vi "csmdoc_export_all_csm_VI_description_doc.vi"(11 "Path":path=path "D:/github/JKI-State-Machine-Plus/.doc/VI Description.md") -> ()   [LabVIEW 2017]
uses:
  Communicable State Machine.lvlib
panel:
  in  "Error in":errorcluster caption="Error in (no error)"
  out "error out":errorcluster
  out "Array":path[](array[path])
  out "concatenated string":string
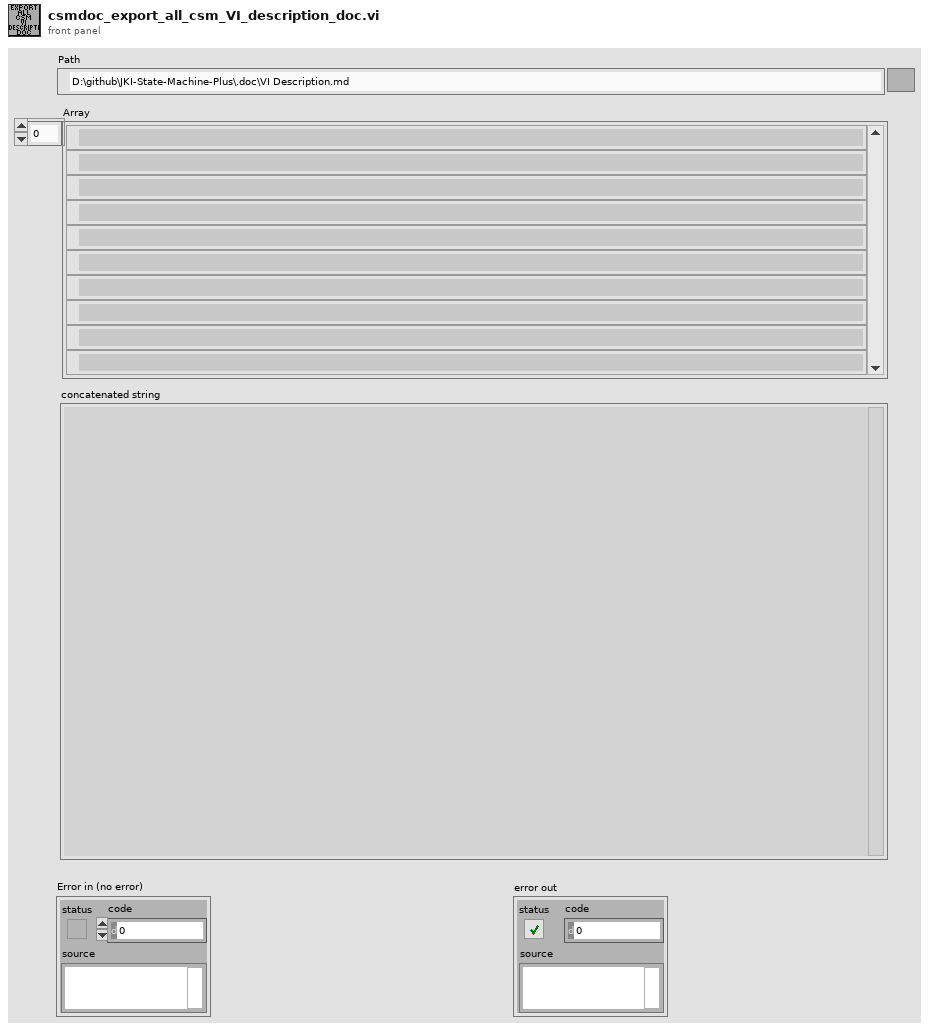
[diagram p1: front panel]
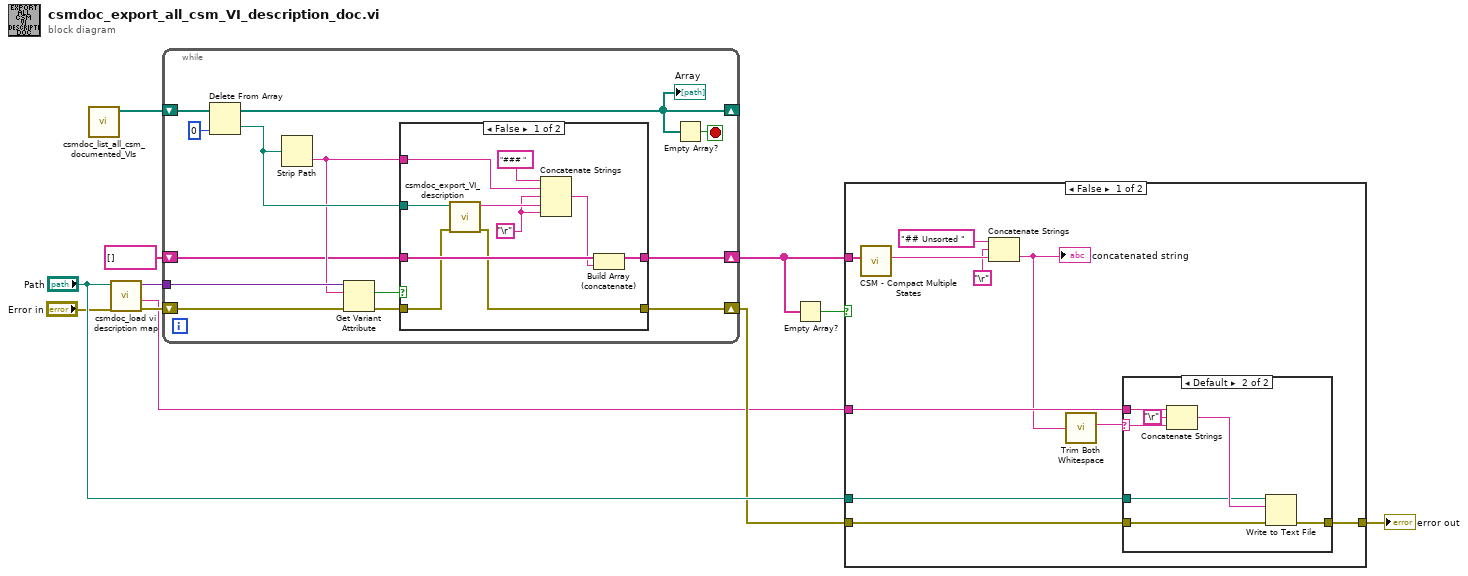
[diagram p0: block diagram]
diagram:
  n1 = call "csmdoc_list_all_csm_documented_VIs.vi"() -> ("Array"=w11:path[])  [unwired: 11 in]
  n2 = call "csmdoc_load vi description map.vi"("Error in"="Error in", "Path"="Path") -> ("Error out"=w7:errorcluster, "text"=w5:string, "variant"=w10:variant)  [unwired: 7 in]
  n3 = while {
    shift-right: [w21] -> _
    shift-left: w11 -> [w23]
    tunnel: w10 -> [w19]
    shift-right: [w16] -> w2
    shift-left: string[] [] -> [w15]
    shift-right: [w12] -> w6
    shift-left: w7 -> [w14]
    stop <- w22 stop-if-true
    n4 = Delete From Array(array=w23, index=0) -> (deleted portion=w24:path, array with subset deleted=w21:path[])  [unwired: 1 in]
    "Array" <- w21
    n5 = Strip Path(path=w24) -> (name=w18:string)  [unwired: 1 out]
    n6 = Get Variant Attribute(Variant=w19, name=w18, error in=w14) -> (found=w17:bool, error out=w13:errorcluster)  [unwired: 1 in, 2 out]
    n7 = case shown="False" w17 {
      tunnel: w24 -> [w31 _]
      tunnel: w18 -> [w30 _]
      tunnel: [w28 w36] -> w16
      tunnel: w15 -> [w29 w36]
      tunnel: w13 -> [w26 w35]
      tunnel: [w25 w35] -> w12
      frame False {
        w32 = "\r"
        n8 = call "csmdoc_export_VI_description.vi"("error in (no error)"=w26, "Path"=w31) -> ("error out"=w25:errorcluster, "concatenated string"=w34:string)  [unwired: 8 in]
        n9 = Concatenate Strings("### " ("string"), w30, w32, w34, w32) -> (w27:string)
        n10 = Build Array (concatenate)(w29, w27) -> (w28:string[])
      }
      frame True {
      }
    }
    n11 = Empty Array?(array=w21) -> (empty?=w22:bool)
  }
  n12 = Empty Array?(array=w2) -> (empty?=w1:bool)
  n13 = case shown="False" w1 {
    tunnel: "Path" -> [w42 _]
    tunnel: w6 -> [w41 w55]
    tunnel: w5 -> [w40 _]
    tunnel: [w38 w55] -> w4
    tunnel: w2 -> [w37 _]
    frame False {
      n14 = call "CSM - Compact Multiple States.vi"("Multiple States"=w37) -> ("States"=w45:string)  [unwired: 9 in]
      n15 = Concatenate Strings("## Unsorted " ("string"), "\r" ("Carriage Return Constant"), w45) -> (w39:string)
      "concatenated string" <- w39
      n16 = call "Trim Both Whitespace.vi"("string"=w39) -> ("trimmed string"=w43:string)  [unwired: 1 in]
      n17 = case shown="Default" w43 {
        selector: w43 -> [_ w53]
        tunnel: w40 -> [_ w52]
        tunnel: w42 -> [_ w50]
        tunnel: w41 -> [w47 w49]
        tunnel: [w47 w48] -> w38
        frame "" {
        }
        frame Default {
          n18 = Concatenate Strings(w52, "\r", w53) -> (w51:string)
          n19 = Write to Text File(file (use dialog)=w50, text=w51, error in=w49) -> (error out=w48:errorcluster)  [unwired: 1 in, 2 out]
        }
      }
    }
    frame True {
    }
  }
  "error out" <- w4
